vi "Local var speed Test.vi"() -> ()   [LabVIEW 2021]
uses:
  Source/Omni-Bus/Omni_Bus.lvclass
  Source/Local Vars/Local Vars.lvclass
  Source/Omni-Bus/Support/Broad Types.ctl
  <vilib>/TSA/Abstract Data Classes/Constants/Support/Str/Str.vi
  <vilib>/TSA/Abstract Data Classes/Constants/Support/Str/Const_Str.lvclass
  <vilib>/TSA/Abstract Data Classes/Constants/Support/DBL/DBL.vi
  <vilib>/TSA/Abstract Data Classes/Constants/Support/DBL/Const_DBL.lvclass
  <vilib>/TSA/Abstract Data Classes/Constants/Support/Bool/Bool.vi
  <vilib>/TSA/Abstract Data Classes/Constants/Support/Bool/Const_Bool.lvclass
  <vilib>/TSA/Abstract Data Classes/Constants/Support/I32/I32.vi
  <vilib>/TSA/Abstract Data Classes/Constants/Support/I32/Const_I32.lvclass
  <vilib>/TSA/Abstract Data Classes/Abs_Types/Type/Abs_Type.lvclass
  <vilib>/TSA/Abstract Data Classes/Abs_Types/Boolean/Abs_Boolean.lvclass
  C:/Program Files (x86)/National Instruments/LabVIEW 2021/vi.lib/TSA/Abstract Data Classes/Abs_Types/Type/Abs_Type.lvclass
  <vilib>/TSA/Abstract Data Classes/Abs_Types/String/Abs_String.lvclass
  <vilib>/TSA/Abstract Data Classes/Abs_Types/I32 Integer/Abs_I32 Integer.lvclass
  C:/Users/Tim/Documents/GitHub/MultiBus/Source/Bus_Access/Bus_Access.lvclass
  <vilib>/TSA/Abstract Data Classes/Abs_Types/Double Float/Support/Type.ctl
  <vilib>/TSA/Abstract Data Classes/Abs_Types/Double Float/Abs_Double Float.lvclass
panel:
  out "error out":errorcluster
  out "x-y":dbl
  out "Value":T1
  out "Tags":string[](array[string])
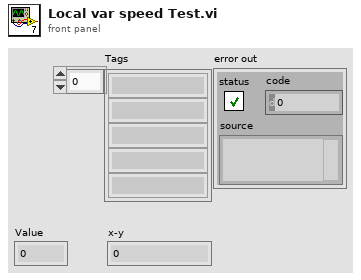
[diagram p1: front panel]
types:
  T1 = typedef "Abs_Double Float.lvclass/Type.ctl" = dbl
  T2 = typedef "Omni_Bus.lvclass/Broad Types.ctl" = enum16{"All Tags", "NI Specific Type", "Boolean", "String", "Numeric", "Float", "Integer", "Collection", "All Value Types", "Non Value Types"}
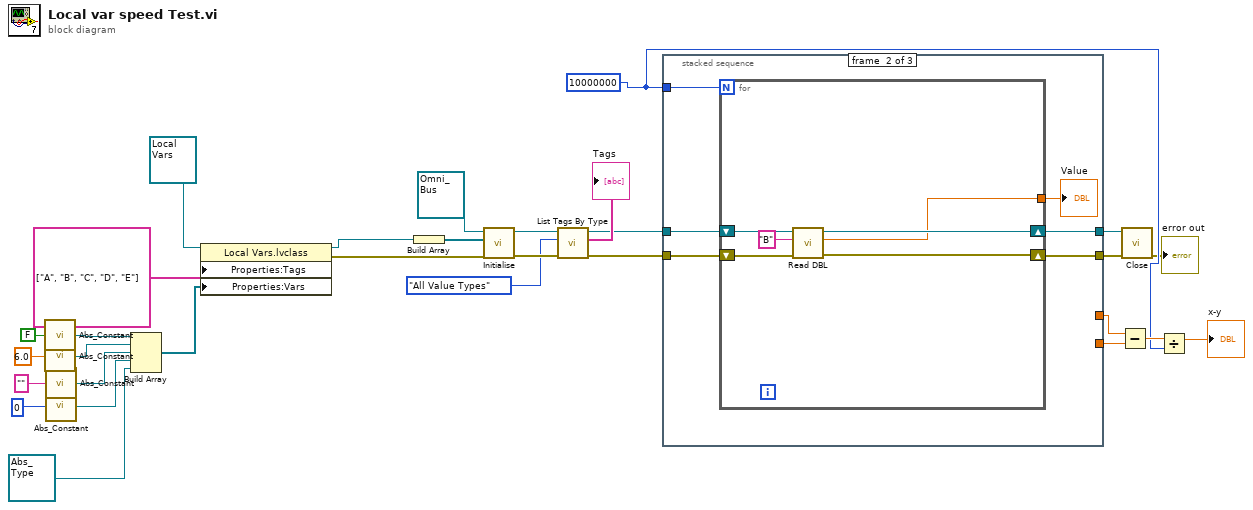
[diagram p0: block diagram]
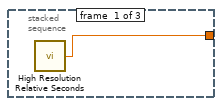
[diagram p2: hidden frame]
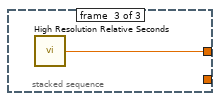
[diagram p3: hidden frame]
diagram:
  w3 = 10000000
  n1 = call-poly <vilib>:"Abs_Constant.vi"("Boolean"=FALSE) -> ("Abs_Boolean.lvclass"=w24:refnum<class "Abs_Boolean.lvclass">)  [unwired: 4 in]
  n2 = call-poly <vilib>:"Abs_Constant.vi"("Value"=6.0) -> ("Constant"=w23:refnum<class "Const_DBL.lvclass">)  [unwired: 4 in]
  n3 = call-poly <vilib>:"Abs_Constant.vi"("String"="") -> ("Abs_String.lvclass"=w22:refnum<class "Abs_String.lvclass">)  [unwired: 4 in]
  n4 = call-poly <vilib>:"Abs_Constant.vi"("Value"=0) -> ("Constant"=w14:refnum<class "Abs_I32 Integer.lvclass">)  [unwired: 4 in]
  n5 = Build Array(w24, w23, w22, w14, refnum<class "Abs_Type.lvclass"> refnum ("Abs_Type.lvclass")) -> (w19:refnum<class "Abs_Type.lvclass">[])
  n6 = property class="Local Vars.lvclass"(reference=refnum<class "Local Vars.lvclass"> refnum ("Data in"), "Properties:Tags"=string[] ["A", "B", "C", "D", "E"] ("Tags"), "Properties:Vars"=w19) -> (reference out=w27:refnum<class "Local Vars.lvclass">, error out=w28:errorcluster)  [unwired: 1 in]
  n7 = Build Array(w27) -> (w29:refnum<class "Local Vars.lvclass">[])
  n8 = call-dynamic "Initialise.vi"("error in (no error)"=w28, "Var Access"=w29, "Var Bus in"=refnum<class "Omni_Bus.lvclass"> refnum) -> ("error out"=w17:errorcluster, "Var Bus out"=w18:refnum<class "Omni_Bus.lvclass">)  [unwired: 7 in]
  n9 = call-dynamic "List Tags By Type.vi"("error in (no error)"=w17, "Broad Types"=Broad_Types."All Value Types", "Var Bus in"=w18) -> ("error out"=w10:errorcluster, "Tags"=→"Tags":string[], "Var Bus out"=w11:refnum<class "Omni_Bus.lvclass">)  [unwired: 5 in, 1 out]
  n10 = stacked-sequence {
    tunnel: w11 -> [_ w37 _]
    tunnel: w10 -> [_ w36 _]
    tunnel: [_ w35 _] -> w9
    tunnel: [_ w34 _] -> w8
    tunnel: [_ _ w44] -> w7
    tunnel: [w31 _ _] -> w6
    tunnel: w3 -> [_ w32 _]
    frame #0 {
      n11 = call <vilib>:"High Resolution Relative Seconds.vi"() -> ("relative seconds"=w31:dbl)
    }
    frame #1 {
      n12 = for {
        N: w32 -> [_]
        shift-right: [w42] -> w35
        shift-left: w37 -> [w43]
        shift-right: [w40] -> w34
        shift-left: w36 -> [w41]
        tunnel: [w39] -> w33
        n13 = call "Read DBL.vi"("error in (no error)"=w41, "Tag"="B", "Var Bus in"=w43) -> ("error out"=w40:errorcluster, "Numeric"=w39:dbl, "Var Bus out"=w42:refnum<class "Omni_Bus.lvclass">)  [unwired: 6 in]
      }
      "Value" <- w33
    }
    frame #2 {
      n14 = call <vilib>:"High Resolution Relative Seconds.vi"() -> ("relative seconds"=w44:dbl)
    }
  }
  n15 = Subtract(x=w7, y=w6) -> (x-y=w5:dbl)
  n16 = call-dynamic "Close.vi"("error in (no error)"=w8, "Data in"=w9) -> ("error out"=→"error out":errorcluster)  [unwired: 8 in, 1 out]
  n17 = Divide(x=w5, y=w3) -> (x/y=→"x-y":dbl)
